vi "CSMP-Sync Call.vi"(0 "state":string, 1 "args":string, 2 "source/target":string, 5 "Error in":errorcluster caption="Error in (no error)", 7 "Response Timeout(5000ms)":i32, 8 "Module Name":string) -> (14 "state out":string, 15 "args out":string, 16 "source/target out":string, 17 "Pre-State out":string, 18 "Pre-Args out":string, 19 "error":errorcluster)   [LabVIEW 2020, in "Communicable State Machine.lvlib"]
uses:
  Communicable State Machine.lvlib
  _Cross CSM State Response.ctl
  _CSM_MSG_TYPE.ctl
  _Cross CSM State Data.ctl
  _CSM_Response Source Message.ctl
  Priority Queue.lvclass/Priority Queue.ctl
  Enqueue Element.vi
  _CSMOFGV.vi
  CSM Not Allowed Message.vi
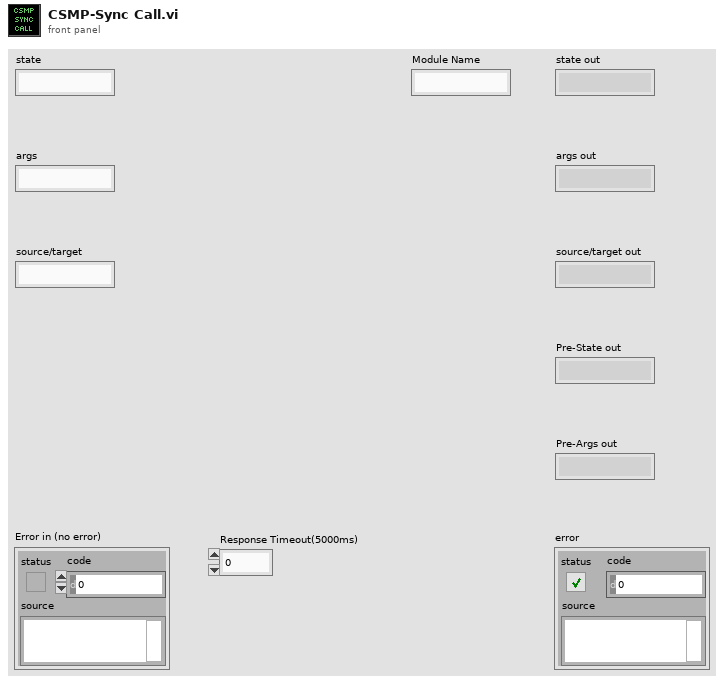
[diagram p1: front panel]
types:
  T1 = typedef "Communicable State Machine.lvlib/_CSMObj.ctl" = cluster{"Requested Name":string, "Module Name":string, "Mode":T2, "Queue":refnum<class "Priority Queue.lvclass">, "CSM-Data":refnum<data-value>, "User Event":refnum<user-event>, "Status Change Event":refnum<user-event>, "Allowed Messages":string[], "Mode-Data":refnum<data-value>, "Group Name":string, "Exit Event":refnum<user-event>}
  T2 = typedef "Communicable State Machine.lvlib/_CSM_MODE.ctl" = enum16{"Not Exist", "Stand Alone", "CSM", "Worker Agent", "Worker", "Chain", "Chain Node"}
  T3 = typedef "Communicable State Machine.lvlib/_Cross CSM State Response.ctl" = cluster{"error":errorcluster, "Response Data":string, "From Who":string}
  T4 = typedef "Communicable State Machine.lvlib/_CSM_MSG_TYPE.ctl" = enum16{"Sync Message(-@)", "Async Message(->)", "Async without Response(->|)", "Async Response", "Broadcast(-><all>)", "Broadcast(-><status>)", "Broadcast(-><interrupt>)", "Append to JKISM States", "Append to JKISM States(High Priority)"}
  T5 = typedef "Communicable State Machine.lvlib/_Cross CSM State Data.ctl" = cluster{"Msg Type":T4, "state":string, "args":string, "source":string, "RespQ":refnum<queue>, "Response For Message":T6, "Target":string}
  T6 = typedef "Communicable State Machine.lvlib/_CSM_Response Source Message.ctl" = cluster{"‘State":string, "’Arguments":string, "’Error":errorcluster}
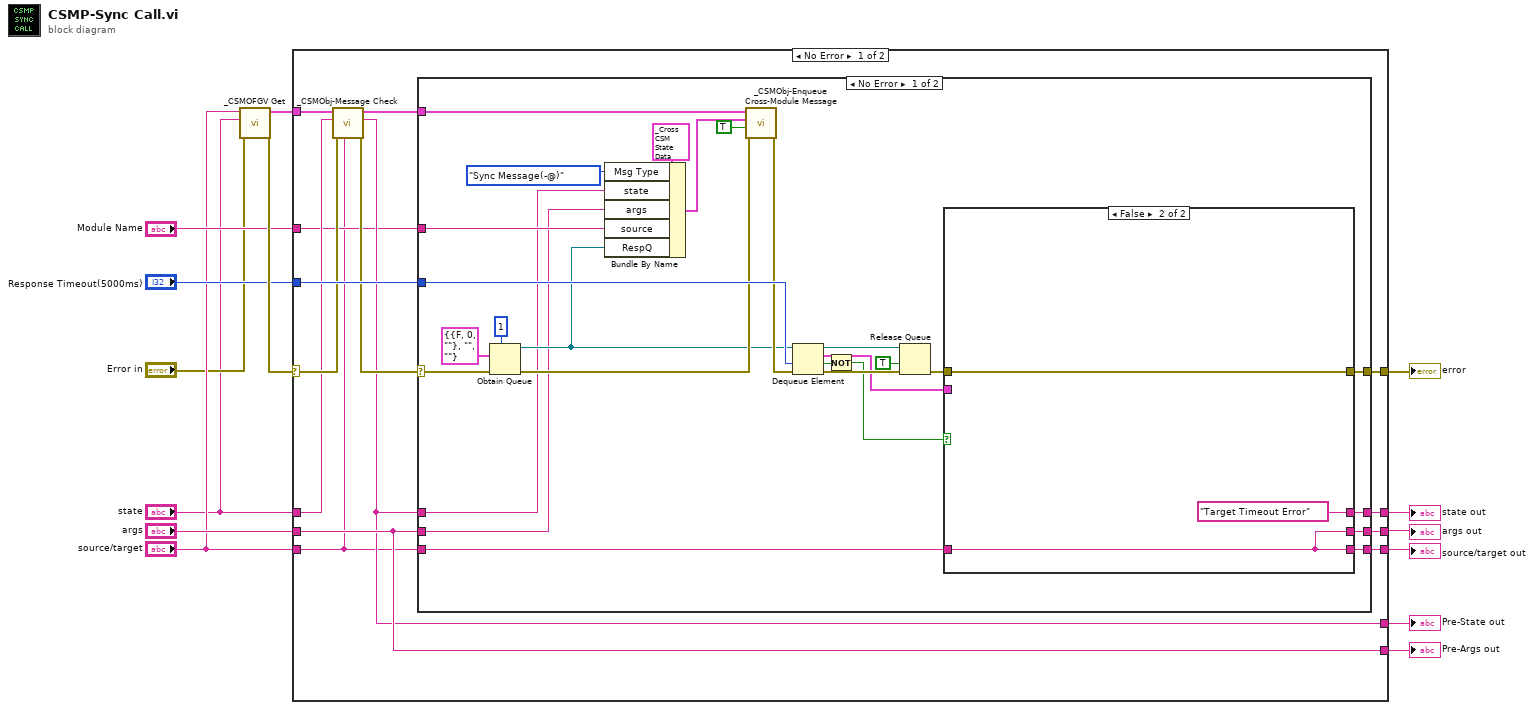
[diagram p0: block diagram]
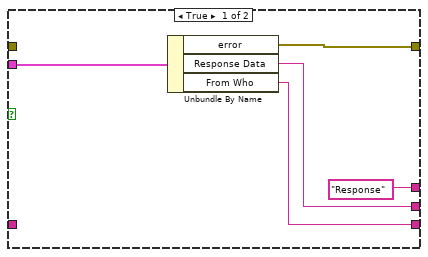
[diagram p2: hidden frame]
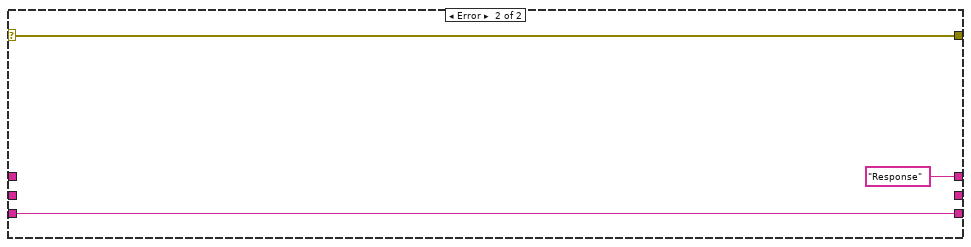
[diagram p3: hidden frame]
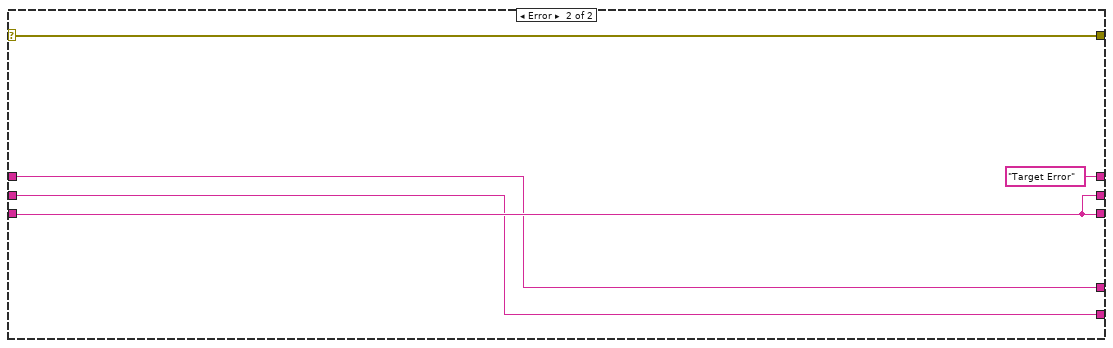
[diagram p4: hidden frame]
diagram:
  n1 = call "_CSMOFGV Get.vi"("Error in"="Error in", "Message"="state", "Name(\"\" to use uuid) in"="source/target") -> ("Error out"=w13:errorcluster, "CSM-Obj"=w14:T1)  [unwired: 6 in, 1 out]
  n2 = case shown="No Error" w13 {
    selector: w13 -> [w20 w70]
    tunnel: "Response Timeout(5000ms)" -> [w28 _]
    tunnel: w14 -> [w22 _]
    tunnel: [w27 "Target Error" ("before match")] -> w8
    tunnel: [w26 w69] -> w7
    tunnel: "source/target" -> [w15 w69]
    tunnel: "state" -> [w18 w68]
    tunnel: "args" -> [w23 w67]
    tunnel: "Module Name" -> [w16 _]
    tunnel: [w23 w67] -> w5
    tunnel: [w25 w70] -> w4
    tunnel: [w17 w68] -> w6
    tunnel: [w24 w69] -> w2
    frame No Error {
      n3 = call "_CSMObj-Message Check.vi"("CSM"=w15, "Error in"=w20, "message"=w18, "CSMQ in"=w22) -> ("Error out"=w19:errorcluster, "message(dup)"=w17:string, "CSMQ out"=w21:T1)  [unwired: 5 in]
      n4 = case shown="No Error" w19 {
        selector: w19 -> [w31 w66]
        tunnel: w28 -> [w55 _]
        tunnel: [w54 "Response" ("f")] -> w27
        tunnel: [w44 _] -> w26
        tunnel: w16 -> [w41 _]
        tunnel: w15 -> [w40 w64]
        tunnel: [w36 w66] -> w25
        tunnel: [w35 w64] -> w24
        tunnel: w23 -> [w34 _]
        tunnel: w21 -> [w32 _]
        tunnel: w17 -> [w30 _]
        frame No Error {
          n5 = Obtain Queue(max queue size (-1, unlimited)=1, element data type=T3 {"error"={"status"=FALSE, "code"=0, "source"=""}, "Response Data"="", "From Who"=""} ("Cross JKI State Machine Response"), error in (no error)=w31) -> (queue out=w43:refnum<queue>, error out=w46:errorcluster)  [unwired: 2 in, 1 out]
          n6 = Bundle By Name(cluster=T5 {"Msg Type"=enum."Sync Message(-@)", "state"="", "args"="", "source"="", "RespQ"=refnum, "Response For Message"={"‘State"="", "’Arguments"="", "’Error"={"status"=FALSE, "code"=0, "source"=""}}, "Target"=""} ("Cross JKI State Machine State"), "Msg Type"=_CSM_MSG_TYPE."Sync Message(-@)", "state"=w30, "args"=w34, "source"=w41, "RespQ"=w43) -> (w50:T5)
          n7 = call "_CSMObj-Enqueue Cross-Module Message.vi"("Error in"=w46, "High Priority?(F)"=TRUE, "Data"=w50, "CSMQ in"=w32) -> ("Error out"=w47:errorcluster)  [unwired: 6 in, 1 out]
          n8 = Dequeue Element(queue=w43, timeout in ms (-1)=w55, error in (no error)=w47) -> (queue out=w49:refnum<queue>, element=w45:T3, timed out?=w53:bool, error out=w48:errorcluster)
          n9 = Not(x=w53) -> (.not. x?=w39:bool)
          n10 = Release Queue(queue=w49, force destroy? (F)=TRUE, error in (no error)=w48) -> (error out=w33:errorcluster)  [unwired: 2 out]
          n11 = case shown="False" w39 {
            tunnel: ["Response" ("f") "Target Timeout Error" ("before match")] -> w54
            tunnel: w45 -> [w60 _]
            tunnel: [w57 w61] -> w44
            tunnel: w40 -> [_ w61]
            tunnel: [w59 w62] -> w36
            tunnel: [w56 w61] -> w35
            tunnel: w33 -> [_ w62]
            frame True {
              n12 = Unbundle By Name(w60) -> ("error"=w59:errorcluster, "Response Data"=w57:string, "From Who"=w56:string)
            }
            frame False {
            }
          }
        }
        frame Error {
        }
      }
    }
    frame Error {
    }
  }
  "state out" <- w8
  "args out" <- w7
  "source/target out" <- w2
  "Pre-State out" <- w6
  "Pre-Args out" <- w5
  "error" <- w4
